vi "ep_Filter and Decimate.vi"(7 "reset? (F)":bool, 8 "error in (no error)":errorcluster, 10 "parameters":T1, 11 "data in":dbl[](array[numeric])) -> (0 "error out":errorcluster, 2 "dup parameters":T1, 3 "data out":dbl[](array[numeric]))   [LabVIEW 2013, in "NI_EP_Resample_Host.lvlib"]
uses:
  <vilib>/addons/Electrical Power/PQ/Resampling/NI_EP_Resample_Host.lvlib
  <vilib>/addons/Electrical Power/PQ/Resampling/Desktop/subVIs/ep_Parameters.ctl
  <vilib>/Analysis/3filter.llb/FIR Filter (DBL).vi
  <vilib>/Analysis/2dsp.llb/Decimate (continuous, DBL).vi
  <vilib>/Analysis/NI_AALBase.lvlib
  <vilib>/Analysis/NI_AALPro.lvlib
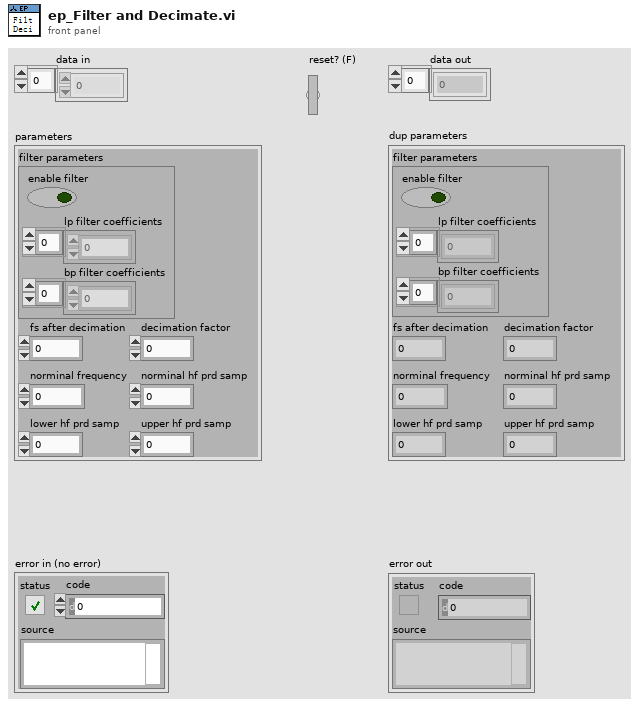
[diagram p1: front panel]
types:
  T1 = typedef "NI_EP_Resample_Host.lvlib/ep_Parameters.ctl" = cluster{"filter parameters":cluster{"enable filter":bool, "lp filter coefficients":dbl[], "bp filter coefficients":dbl[]}, "fs after decimation":dbl, "decimation factor":i32, "norminal frequency":dbl, "norminal hf prd samp":dbl, "lower hf prd samp":i32, "upper hf prd samp":i32}
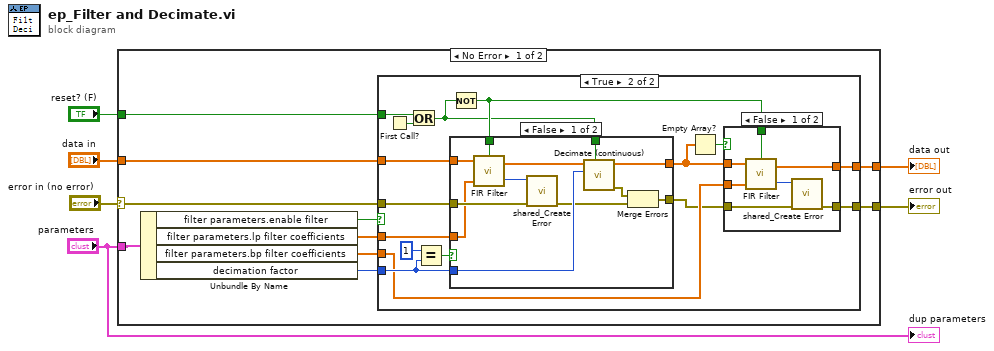
[diagram p0: block diagram]
diagram:
  n1 = case shown="No Error" "error in (no error)" {
    selector: "error in (no error)" -> [w14 w57]
    tunnel: "parameters" -> [w16 _]
    tunnel: "reset? (F)" -> [w15 _]
    tunnel: [w13 w57] -> w4
    tunnel: [w12 _] -> w3
    tunnel: "data in" -> [w8 _]
    frame No Error {
      n2 = Unbundle By Name(w16) -> ("filter parameters.enable filter"=w11:bool, "filter parameters.lp filter coefficients"=w10:dbl[], "filter parameters.bp filter coefficients"=w9:dbl[], "decimation factor"=w7:i32)
      n3 = case shown="True" w11 {
        tunnel: w10 -> [_ w29]
        tunnel: w9 -> [_ w23]
        tunnel: w7 -> [_ w24]
        tunnel: w15 -> [_ w33]
        tunnel: w8 -> [w17 w31]
        tunnel: w14 -> [w18 w30]
        tunnel: [w18 w22] -> w13
        tunnel: [w17 w20] -> w12
        frame False {
        }
        frame True {
          n4 = First Call?() -> (First Call?: T/F=w34:bool)
          n5 = Or(x=w33, y=w34) -> (x .or. y?=w21:bool)
          n6 = Equal?(x=1 ("y"), y=w24) -> (x = y?=w32:bool)
          n7 = Not(x=w21) -> (.not. x?=w26:bool)
          n8 = case shown="False" w32 {
            tunnel: w31 -> [w54 w56]
            tunnel: [w47 w56] -> w27
            tunnel: w30 -> [w52 w55]
            tunnel: w29 -> [w51 _]
            tunnel: w26 -> [w50 _]
            tunnel: w21 -> [w49 _]
            tunnel: w24 -> [w48 _]
            tunnel: [w45 w55] -> w19
            frame False {
              n9 = call-poly <vilib>:"FIR Filter.vi"("init/cont (init:F)"=w50, "FIR Coefficients"=w51, "X"=w54) -> ("error"=w53:i32, "Filtered X"=w46:dbl[])  [unwired: 1 in]
              n10 = call <vilib>:"shared_Create Error.vi"("error in (no error)"=w52, "error code (0)"=w53) -> ("error out"=w43:errorcluster)  [unwired: 9 in]
              n11 = call-poly <vilib>:"Decimate (continuous).vi"("reset"=w49, "decimating factor"=w48, "X"=w46) -> ("error out"=w44:errorcluster, "Decimated Array"=w47:dbl[])  [unwired: 7 in]
              n12 = Merge Errors(w44, w43) -> (w45:errorcluster)
            }
            frame True {
            }
          }
          n13 = Empty Array?(array=w27) -> (empty?=w28:bool)
          n14 = case shown="False" w28 {
            tunnel: w27 -> [w41 _]
            tunnel: [w40 _] -> w20
            tunnel: w26 -> [w39 _]
            tunnel: w19 -> [w38 w42]
            tunnel: [w36 w42] -> w22
            tunnel: w23 -> [w35 _]
            frame False {
              n15 = call-poly <vilib>:"FIR Filter.vi"("init/cont (init:F)"=w39, "FIR Coefficients"=w35, "X"=w41) -> ("error"=w37:i32, "Filtered X"=w40:dbl[])  [unwired: 1 in]
              n16 = call <vilib>:"shared_Create Error.vi"("error in (no error)"=w38, "error code (0)"=w37) -> ("error out"=w36:errorcluster)  [unwired: 9 in]
            }
            frame True {
            }
          }
        }
      }
    }
    frame Error {
    }
  }
  "error out" <- w4
  "data out" <- w3
  "dup parameters" <- "parameters"
